vi "Read NET_StreamCancellationSource.vi"(8 "error in (no error)":errorcluster, 11 "HttpContent in":refnum<class "HttpContent.lvclass">) -> (0 "error out":errorcluster, 2 "NET_CancellationSource":refnum<k24>, 3 "HttpContent out":refnum<class "HttpContent.lvclass">)   [LabVIEW 2018, in "HttpClient_NET.lvlib" / "HttpContent.lvclass"]
doc: "<b> </b> <b> </b>\nHttpClient_NET\nJustin Young - Viviota\nCopyright (c) 2021\nLicense: BSD"
uses:
  HttpContent.lvclass
  HttpContent.lvclass/HttpContent.ctl
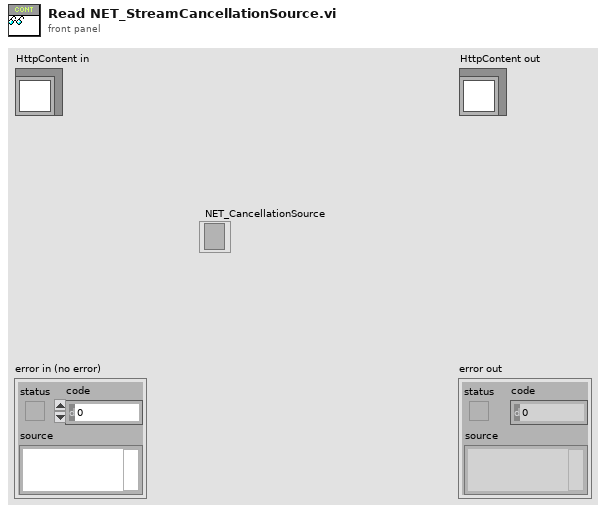
[diagram p1: front panel]
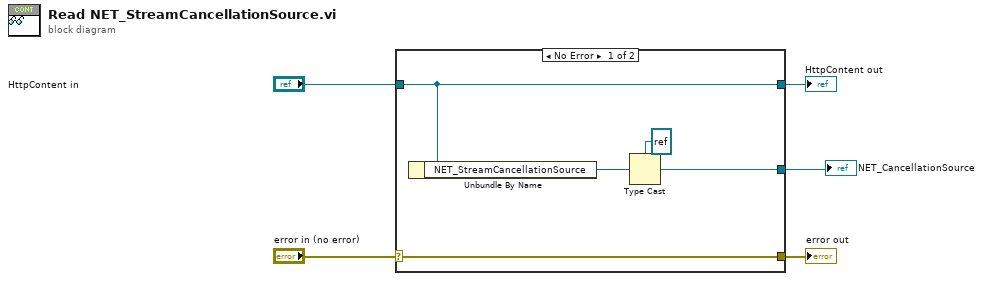
[diagram p0: block diagram]
diagram:
  n1 = case shown="No Error" "error in (no error)" {
    selector: "error in (no error)" -> [w10 w11]
    tunnel: [w10 w11] -> w4
    tunnel: [w9 w12] -> w2
    tunnel: "HttpContent in" -> [w9 w12]
    tunnel: [w7 _] -> w1
    frame No Error {
      n2 = Unbundle By Name(w9) -> ("NET_StreamCancellationSource"=w8:i64)
      n3 = Type Cast(type=refnum<k24> refnum ("NET_CancellationSource"), x=w8) -> (*(type *) &x=w7:refnum<k24>)
    }
    frame Error {
    }
  }
  "error out" <- w4
  "HttpContent out" <- w2
  "NET_CancellationSource" <- w1
